vi "rot - Givens Rotation.vi"   [LabVIEW 2020, in "NI_AALBLAS.lvlib"]
doc: "Applies a Givens rotation to a set of points."
uses:
  NI_AALBLAS.lvlib
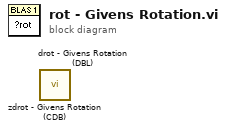
[diagram p0: block diagram]
diagram:
  n1 = call "zdrot - Givens Rotation (CDB).vi"() -> ()  [unwired: 9 in, 3 out]
  n2 = call "drot - Givens Rotation (DBL).vi"() -> ()  [unwired: 9 in, 3 out]
